vi "Get_coords_from_bounding_box.vi"(2 "Error In":errorcluster, 3 "Object Bounding Box":T1) -> (0 "Error Out":errorcluster, 1 "Object Coords (center)":cluster{"X":dbl, "Y":dbl})   [LabVIEW 2018, in "Cage Diagram.lvlib"]
uses:
  Cage Diagram.lvlib
  <vilib>/Analysis/baseanly.llb/Mean (DBL).vi
  <vilib>/Analysis/NI_AALBase.lvlib
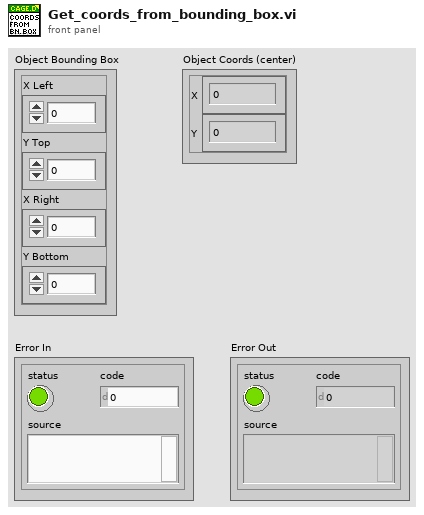
[diagram p1: front panel]
types:
  T1 = cluster{"X Left":dbl, "Y Top":dbl, "X Right":dbl, "Y Bottom":dbl}
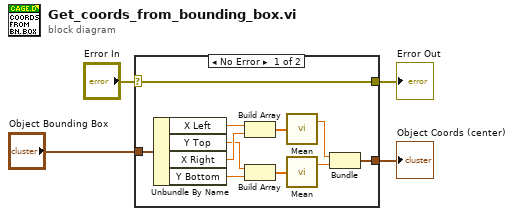
[diagram p0: block diagram]
diagram:
  n1 = case shown="No Error" "Error In" {
    selector: "Error In" -> [w15 w16]
    tunnel: [w15 w16] -> w3
    tunnel: "Object Bounding Box" -> [w14 _]
    tunnel: [w5 _] -> w1
    frame No Error {
      n2 = Unbundle By Name(w14) -> ("X Left"=w13:dbl, "Y Top"=w9:dbl, "X Right"=w12:dbl, "Y Bottom"=w8:dbl)
      n3 = Build Array(w13, w12) -> (w11:dbl[])
      n4 = Build Array(w9, w8) -> (w10:dbl[])
      n5 = call-poly <vilib>:"Mean.vi"("X"=w11) -> ("mean"=w7:dbl)  [unwired: 1 out]
      n6 = call-poly <vilib>:"Mean.vi"("X"=w10) -> ("mean"=w6:dbl)  [unwired: 1 out]
      n7 = Bundle("mean"=w7, "mean"=w6) -> (w5:cluster{"mean":dbl, "mean":dbl})  [unwired: 1 in]
    }
    frame Error {
    }
  }
  "Error Out" <- w3
  "Object Coords (center)" <- w1
